vi "DataBinding-transmitter.vi"() -> ()   [LabVIEW 2020]
uses:
  <vilib>/numeric/Random Number (Range) I64.vi
  <vilib>/numeric/sub_Random U32.vi
panel:
  out "Waveform Chart":i64(graph)
  out "Gauge":dbl(knob) scale=0.0..100.0
  out "sent item":i64
  in  "stop":bool
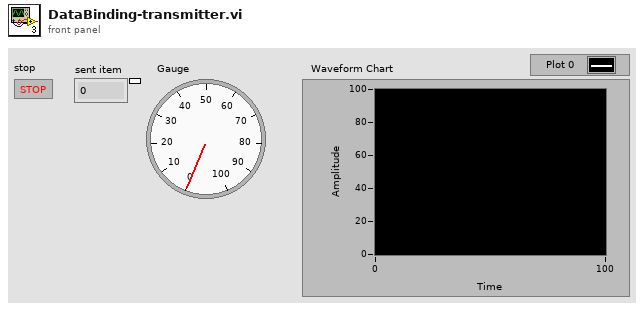
[diagram p1: front panel]
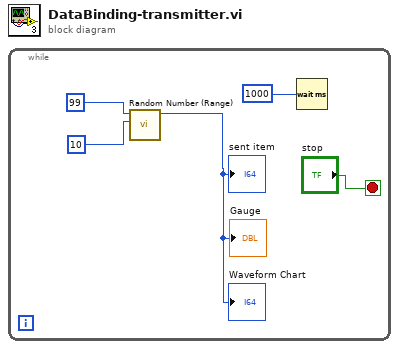
[diagram p0: block diagram]
diagram:
  n1 = while {
    stop <- "stop" stop-if-true
    n2 = call-poly <vilib>:"Random Number (Range).vi"("lower bound (-100)"=10, "upper bound (100)"=99) -> ("number"=→"sent item" →"Gauge" →"Waveform Chart":i64)  [unwired: 9 in]
    n3 = Wait (ms)(milliseconds to wait=1000) -> ()  [unwired: 1 out]
  }
